vi "UmlFileOpener_20XX.vi"() -> ()   [LabVIEW 2014]
uses:
  <vilib>/Utility/miscctls.llb/LVRectTypeDef.ctl
panel:
  out "Port":i32
  out "error out":errorcluster
  out "resulting string":string
  out "Application:Command Line Arguments":string[](array[string])
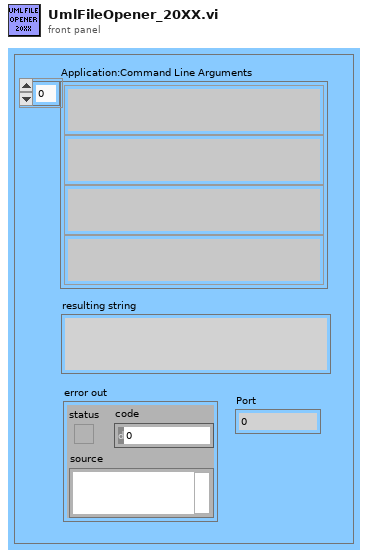
[diagram p1: front panel]
types:
  T1 = enum32{"invalid OS target", "Mac OS", "Windows 3.1", "Windows 95/NT", "Solaris 1", "Solaris 2", "HP-UX", "PowerMAX", "Linux", "Irix", "Rhapsody", "BeOS", "AIX", "OSF1", "VxWorks", "PharLap", "Carbon", "RTX", "Windows x64", "Linux x64"}
  T2 = enum32{"invalid app kind", "Development System", "Run Time System", "Student Edition", "Embedded LabVIEW", "Evaluation", "Custom"}
  T3 = typedef "LVRectTypeDef.ctl" = cluster{"Left":i16, "Top":i16, "Right":i16, "Bottom":i16}
  T4 = enum32{"invalid OS target", "Mac OS", "Windows 3.1", "Windows 95/NT", "Solaris 1", "Solaris 2", "HP-UX", "PowerMAX", "Linux", "Irix", "Rhapsody", "BeOS", "AIX", "OSF1", "VxWorks", "PharLap", "Carbon", "RTX", "Windows x64", "Linux x64", "Mac OS X x64"}
  T5 = enum16{"open", "replace", "create", "open or create", "replace or create", "replace or create with confirmation"}
  T6 = enum16{"OpenUmlEditor", "ReverseEngineering:WholeProject", "ReverseEngineering:OneClass", "ReverseEngineering:OneVI", "ShowInStateDiagram:OneVI", "OpenUMLFile"}
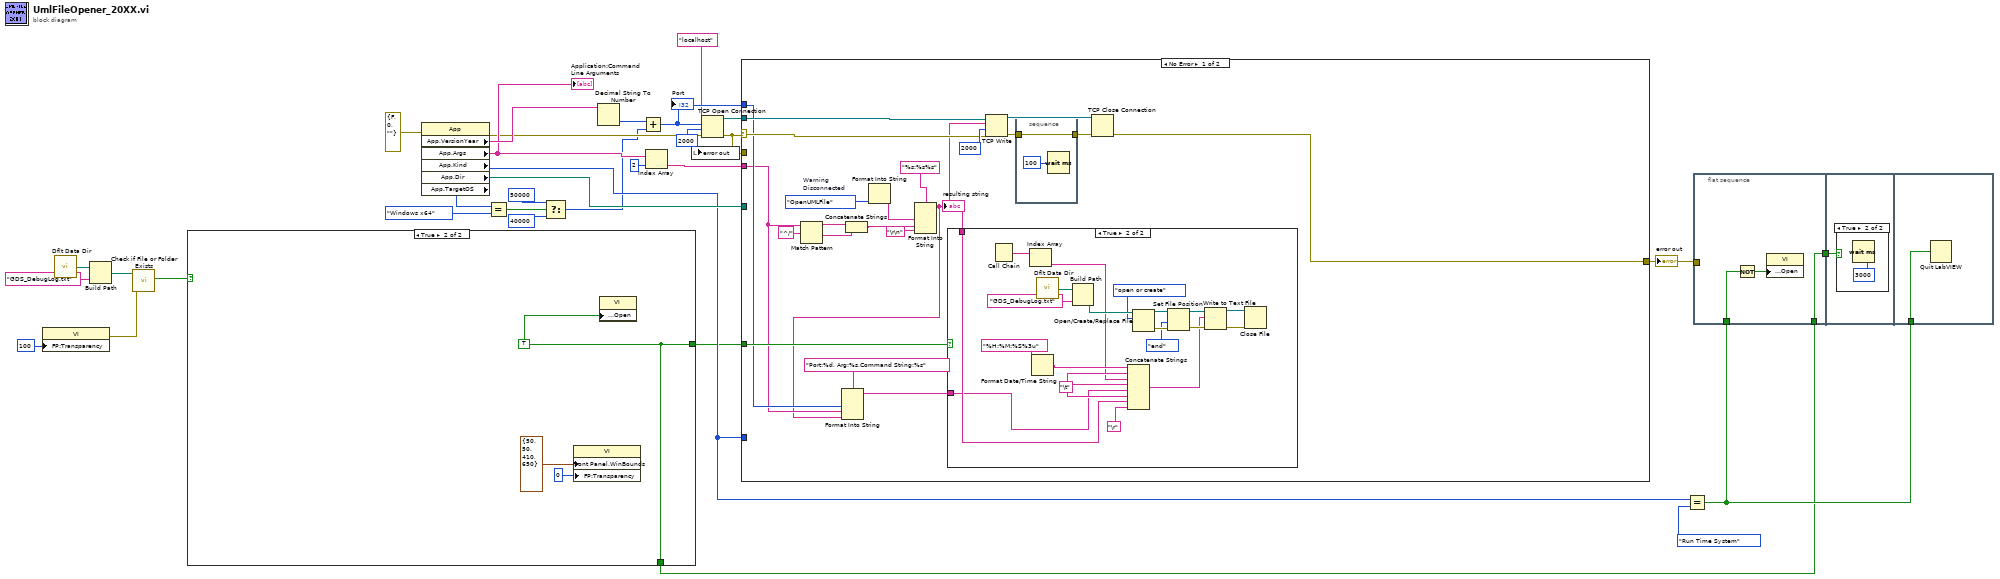
[diagram p0: block diagram]
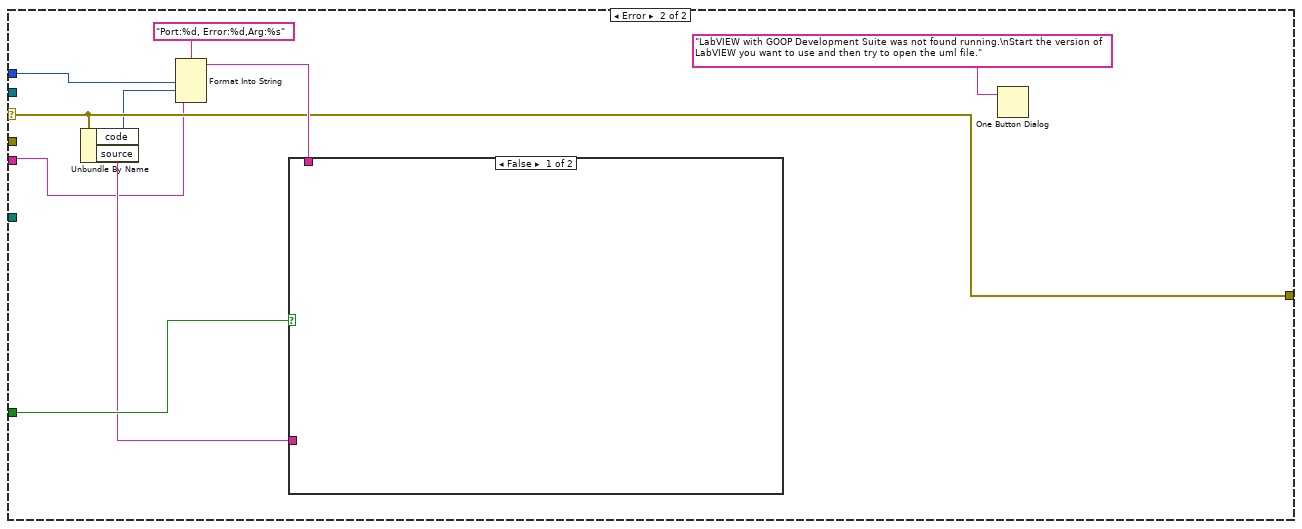
[diagram p4: hidden frame]
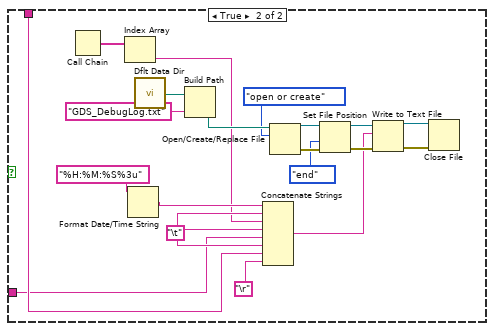
[diagram p5: hidden frame]
diagram:
  n1 = property class="VI"("FP:Transparency"=u8 100 ("Front Panel Window:Transparency")) -> (error out=w7:errorcluster)  [unwired: 2 in, 1 out]
  n2 = call <vilib>:"Dflt Data Dir.vi"() -> ("App:Default Data Directory"=w15:path)
  n3 = Build Path(base path=w15, name or relative path="GDS_DebugLog.txt") -> (appended path=w16:path)
  n4 = call <vilib>:"Check if File or Folder Exists.vi"("error in (no error)"=w7, "path"=w16) -> ("file or folder exists?"=w13:bool)  [unwired: 7 in, 2 out]
  n5 = case shown="True" w13 {
    tunnel: [_ w33] -> w18
    tunnel: [_ w33] -> w12
    frame False {
    }
    frame True {
      w33 = TRUE
      n6 = property class="VI"("Front Panel.WinBounds"=T3 {"Left"=50, "Top"=50, "Right"=410, "Bottom"=650} ("Front Panel Window:Window Bounds"), "FP:Transparency"=u8 0 ("Front Panel Window:Transparency")) -> ()  [unwired: 2 in, 2 out]
      n7 = property class="VI"("Front Panel.Open"=w33) -> ()  [unwired: 2 in, 2 out]
    }
  }
  n8 = property class="App"(error in=errorcluster {"status"=FALSE, "code"=0, "source"=""} ("error in (no error)")) -> (error out=w21:errorcluster, "App.VersionYear"=w30:string, "App.Args"=w24:string[], "App.Kind"=w19:T2, "App.Dir"=w31:path, "App.TargetOS"=w6:T4)  [unwired: 1 in, 1 out]
  "Application:Command Line Arguments" <- w24
  n9 = Equal?(x=w6, y=T1."Windows x64") -> (x = y?=w4:bool)
  n10 = Select(t=50000 ("y"), s=w4, f=40000 ("y")) -> (s? t:f=w1:i32)
  n11 = Decimal String To Number(string=w30) -> (number=w29:i32)  [unwired: 2 in, 1 out]
  n12 = Add(x=w29, y=w1) -> (x+y=w11:i32)
  "Port" <- w11
  n13 = Index Array(array=w24, index=2) -> (element=w23:string)
  n14 = TCP Open Connection(address="localhost", remote port or service name=w11, timeout ms (60000)=2000, error in (no error)=w21) -> (connection ID=w26:refnum<k5>, error out=w10:errorcluster)  [unwired: 1 in]
  n15 = local write "error out"(w10) -> ()
  n16 = case shown="No Error" w10 {
    selector: w10 -> [w42 w82]
    tunnel: [w51 w82] -> w20
    tunnel: w31 -> [_ _]
    tunnel: w26 -> [w43 _]
    tunnel: w23 -> [w38 w79]
    tunnel: w19 -> [_ _]
    tunnel: w12 -> [w41 w86]
    tunnel: w11 -> [w39 w83]
    tunnel: w10 -> [_ _]
    frame No Error {
      w56 = T6."OpenUMLFile"  # Warning Disconnected
      n17 = Match Pattern(string=w38, regular expression="^/") -> (before substring=w49:string, after substring=w48:string)  [unwired: 1 in, 2 out]
      n18 = Concatenate Strings(w49, w48) -> (w47:string)
      n19 = Format Into String(w56) -> (resulting string=w54:string)  [unwired: 3 in, 1 out]
      n20 = Format Into String(format string="%s:%s%s", w54, w47, "\r\n") -> (resulting string=w37:string)  [unwired: 2 in, 1 out]
      "resulting string" <- w37
      n21 = Format Into String(format string="Port:%d, Arg:%s,Command String:%s", w39, w38, w37) -> (resulting string=w36:string)  [unwired: 2 in, 1 out]
      n22 = case shown="True" w41 {
        tunnel: w37 -> [_ w58]
        tunnel: w36 -> [_ w57]
        frame False {
        }
        frame True {
          w60 = "\t"
          n23 = Call Chain() -> (call chain=w62:string[])
          n24 = Index Array(array=w62) -> (element=w59:string)  [unwired: 1 in]
          n25 = Format Date/Time String(time format string (%c)="%H:%M:%S%3u") -> (date/time string=w61:string)  [unwired: 2 in]
          n26 = call <vilib>:"Dflt Data Dir.vi"() -> ("App:Default Data Directory"=w75:path)
          n27 = Build Path(base path=w75, name or relative path="GDS_DebugLog.txt") -> (appended path=w74:path)
          n28 = Concatenate Strings(w61, w60, w59, w60, w57, w60, w58, "\r") -> (w63:string)
          n29 = Open/Create/Replace File(file path (use dialog)=w74, operation (0:open)=T5."open or create") -> (refnum out=w71:refnum<file>, error out=w72:errorcluster)  [unwired: 4 in, 1 out]
          n30 = Set File Position(refnum=w71, from (0:start)=enum16{"start", "end", "current"}."end", error in=w72) -> (refnum out=w68:refnum<file>, error out=w69:errorcluster)  [unwired: 1 in]
          n31 = Write to Text File(file (use dialog)=w68, text=w63, error in=w69) -> (refnum out=w66:refnum<file>, error out=w67:errorcluster)  [unwired: 1 in, 1 out]
          n32 = Close File(refnum=w66, error in=w67) -> ()  [unwired: 2 out]
        }
      }
      n33 = TCP Write(connection ID=w43, data in=w37, error in (no error)=w42, 9:2000 ("timeout ms (25000)")) -> (connection ID out=w52:refnum<k5>, error out=w45:errorcluster)  [unwired: 1 out]
      n34 = stacked-sequence {
        tunnel: w45 -> [w77]
        tunnel: [w77] -> w44
        frame #0 {
          n35 = Wait (ms)(milliseconds to wait=u32 100) -> ()  [unwired: 1 out]
        }
      }
      n36 = TCP Close Connection(connection ID=w52, error in (no error)=w44) -> (error out=w51:errorcluster)  [unwired: 1 in, 1 out]
    }
    frame Error {
      n37 = Unbundle By Name(w82) -> ("code"=w81:i32, "source"=w80:string)
      n38 = Format Into String(format string="Port:%d, Error:%d,Arg:%s", w83, w81, w79) -> (resulting string=w84:string)  [unwired: 2 in, 1 out]
      n39 = case shown="False" w86 {
        tunnel: w84 -> [_ w89]
        tunnel: w80 -> [_ w88]
        frame False {
        }
        frame True {
          w91 = "\t"
          n40 = Call Chain() -> (call chain=w93:string[])
          n41 = Index Array(array=w93) -> (element=w90:string)  [unwired: 1 in]
          n42 = Format Date/Time String(time format string (%c)="%H:%M:%S%3u") -> (date/time string=w92:string)  [unwired: 2 in]
          n43 = call <vilib>:"Dflt Data Dir.vi"() -> ("App:Default Data Directory"=w106:path)
          n44 = Build Path(base path=w106, name or relative path="GDS_DebugLog.txt") -> (appended path=w105:path)
          n45 = Concatenate Strings(w92, w91, w90, w91, w88, w91, w89, "\r") -> (w94:string)
          n46 = Open/Create/Replace File(file path (use dialog)=w105, operation (0:open)=T5."open or create") -> (refnum out=w102:refnum<file>, error out=w103:errorcluster)  [unwired: 4 in, 1 out]
          n47 = Set File Position(refnum=w102, from (0:start)=enum16{"start", "end", "current"}."end", error in=w103) -> (refnum out=w99:refnum<file>, error out=w100:errorcluster)  [unwired: 1 in]
          n48 = Write to Text File(file (use dialog)=w99, text=w94, error in=w100) -> (refnum out=w97:refnum<file>, error out=w98:errorcluster)  [unwired: 1 in, 1 out]
          n49 = Close File(refnum=w97, error in=w98) -> ()  [unwired: 2 out]
        }
      }
      n50 = One Button Dialog(message="LabVIEW with GOOP Development Suite was not found running.\nStart the version of LabVIEW you want to use and then try to open the uml file.") -> ()  [unwired: 1 in, 1 out]
    }
  }
  "error out" <- w20
  n51 = Equal?(x=w19, y=T2."Run Time System") -> (x = y?=w22:bool)
  n52 = flat-sequence {
    tunnel: w20 -> [_]
    tunnel: w22 -> [w110]
    tunnel: w18 -> [w108]
    tunnel: [w108] -> w17
    tunnel: w17 -> [w111]
    tunnel: w22 -> [w113]
    frame #0 {
      n53 = Not(x=w110) -> (.not. x?=w109:bool)
      n54 = property class="VI"("Front Panel.Open"=w109) -> ()  [unwired: 2 in, 2 out]
    }
    frame #1 {
      n55 = case shown="True" w111 {
        frame False {
        }
        frame True {
          n56 = Wait (ms)(milliseconds to wait=u32 3000) -> ()  [unwired: 1 out]
        }
      }
    }
    frame #2 {
      n57 = Quit LabVIEW(quit? (T)=w113) -> ()
    }
  }
